vi "FGV Map Example.vi"() -> ()   [LabVIEW 2020, in "FGV Map.lvlib"]
uses:
  FGV Map.lvlib
  Get Data/FGV Map Get Data (String).vi
panel:
  out "Deleted Data":variant
  out "Data Out":string
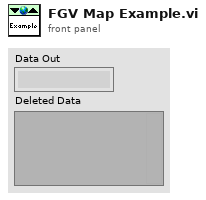
[diagram p1: front panel]
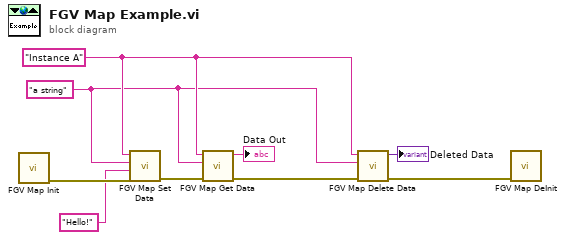
[diagram p0: block diagram]
diagram:
  w3 = "a string" ("Data Key")
  w4 = "Instance A" ("Instance Key")
  n1 = call "FGV Map Init.vi"() -> ("error out"=w9:errorcluster)  [unwired: 11 in]
  n2 = call "FGV Map Set Data.vi"("error in (no error)"=w9, "Data In"="Hello!" ("Data Key"), "Data Key"=w3, "Instance Key"=w4) -> ("error out"=w7:errorcluster)  [unwired: 5 in, 2 out]
  n3 = call-poly "FGV Map Get Data.vi"("error in (no error)"=w7, "Data Key"=w3, "Instance Key"=w4) -> ("error out"=w5:errorcluster, "Data Out"=→"Data Out":string)  [unwired: 6 in, 1 out]
  n4 = call "FGV Map Delete Data.vi"("error in (no error)"=w5, "Data Key"=w3, "Instance Key"=w4) -> ("error out"=w1:errorcluster, "Deleted Data"=→"Deleted Data":variant)  [unwired: 6 in, 1 out]
  n5 = call "FGV Map DeInit.vi"("error in"=w1) -> ()  [unwired: 10 in, 1 out]
